vi "changeVel.vi"(1 "vel (mm/s)":dbl=10.0, 2 "systemIdx":i32, 3 "System no.":i32=1 min=1 max=4 step=1) -> (0 "Controller error":bool)   [LabVIEW 2015]
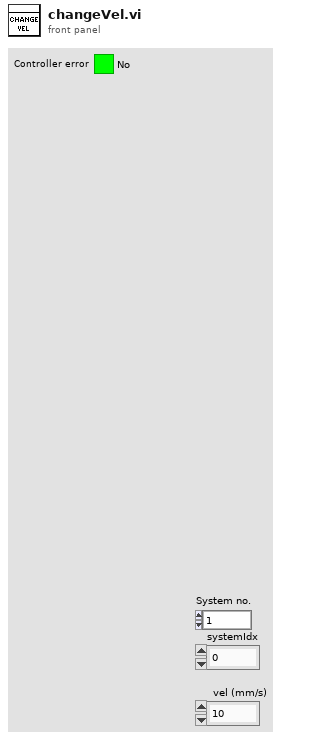
[diagram p1: front panel]
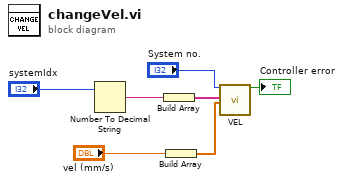
[diagram p0: block diagram]
diagram:
  n1 = Number To Decimal String(number="systemIdx") -> (decimal integer string=w5:string)  [unwired: 1 in]
  n2 = Build Array(w5) -> (w4:string[])
  n3 = Build Array("vel (mm/s)") -> (w6:dbl[])
  n4 = call "VEL.vi"("System no."="System no.", "Axes to set"=w4, "Velocity values"=w6) -> ("Controller error"=→"Controller error":bool)  [unwired: 15 in, 1 out]
